vi "PlungerTEst.vi"() -> ()   [LabVIEW 2011]
uses:
  plungerstatus.ctl
panel:
  in  "Ring":u16(ring)
  out "read switches":T1[](array[typedef])
  in  "Phosphor":bool
  in  "Wedge":bool
  in  "Beam Dump 2":bool
  in  "Beam Dump 1":bool
  out "plunger status":enum16{"ASSERTED", "DE-ASSERTED\nOUT OF BEAM"}[](array[ring])
  in  "stop":bool
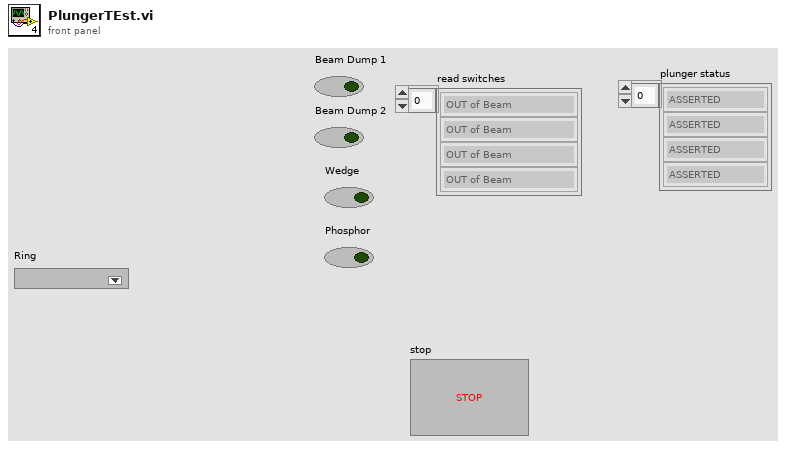
[diagram p1: front panel]
types:
  T1 = typedef "plungerstatus.ctl" = enum16{"unknown", "OUT of Beam", "IN Beam"}
  T2 = enum16{"Beam Dump 1", "Beam Dump 2", "Wedge", "Phosphor"}
  T3 = cluster{"bits 2":bool[], "bits 2":bool[], "bits 2":bool[], i32[]}
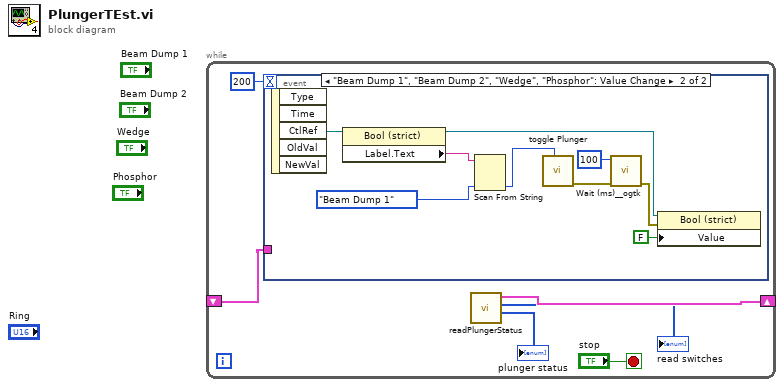
[diagram p0: block diagram]
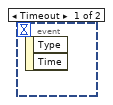
[diagram p2: hidden frame]
diagram:
  n1 = while {
    shift-right: [w4] -> _
    shift-left: _ -> [w3]
    stop <- "stop" stop-if-true
    n2 = event shown="[1] \"Beam Dump 1\", \"Beam Dump 2\", \"Wedge\", \"Phosphor\": Value Change" {
      selector: _ -> [_ _]
      dyn-events: _ -> [_ _]
      timeout: 200 -> [_ _]
      tunnel: w3 -> [_ _]
      event Timeout {
        n3 = event-data() -> ()  [unwired: 1 in, 2 out]
      }
      event "Beam Dump 1", "Beam Dump 2", "Wedge", "Phosphor": Value Change {
        n4 = event-data() -> ("CtlRef"=w15:refnum<vi>)  [unwired: 1 in, 4 out]
        n5 = property class="Bool (strict)"(reference=w15) -> (reference out=w7:refnum<vi>, "Label.Text"=w14:string)  [unwired: 1 in, 1 out]
        n6 = Scan From String(input string=w14, default 1=T2."Beam Dump 1" ("Plunger")) -> (output 1=w12:T2)  [unwired: 3 in, 3 out]
        n7 = call "toggle Plunger.vi"("Plunger"=w12) -> ("error out"=w11:errorcluster)  [unwired: 10 in]
        n8 = call <userlib>:"Wait (ms)__ogtk.vi"("error in (no error)"=w11, "milliseconds to wait"=u32 100) -> ("error out"=w9:errorcluster)  [unwired: 8 in, 1 out]
        n9 = property class="Bool (strict)"(reference=w7, error in=w9, "Value"=FALSE) -> ()  [unwired: 2 out]
      }
    }
    n10 = call "readPlungerStatus.vi"() -> ("plunger status"=→"plunger status":enum16{"ASSERTED", "DE-ASSERTED\nOUT OF BEAM"}[], "read switches"=→"read switches":T1[], "Cluster 3"=w4:T3)  [unwired: 9 in]
  }
